vi "RA_Trigger_HC_SR04 V2.vi"() -> ()   [LabVIEW 2021]
uses:
  <vilib>/Analysis/NI_AALBase.lvlib
panel:
  in  "stop":bool
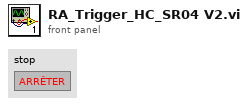
[diagram p1: front panel]
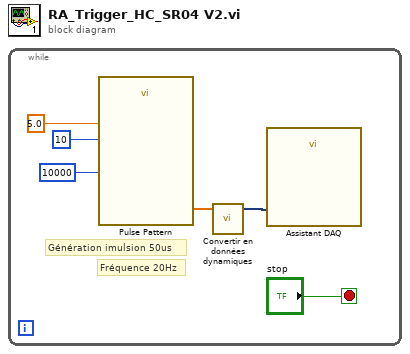
[diagram p0: block diagram]
diagram:
  n1 = while {
    stop <- "stop" stop-if-true
    # "Fréquence 20Hz"
    # "Génération imulsion 50us"
    n2 = call <vilib>:"Pulse Pattern.vi"("width"=10, "amplitude"=5.0, "samples"=10000) -> ("Pulse Pattern"=w1:dbl[])  [unwired: 1 in, 1 out]
    n3 = call "Convertir en données dynamiques"("Array"=w1) -> ("Dynamic Data Type"=w6:dynamicdata)  [unwired: 3 in]
    n4 = call "Assistant DAQ"("data"=w6) -> ()  [unwired: 16 in, 3 out]
  }
